vi "Proceed Directory.vi"(8 "error in (no error)":errorcluster, 9 "path":path, 10 "Load Image Report":bool, 11 "Launch File Viewer in":refnum<class "HIJ Vision File Viewer App.lvclass">) -> (0 "error out":errorcluster, 3 "Launch File Viewer out":refnum<class "HIJ Vision File Viewer App.lvclass">)   [LabVIEW 2014, in "HIJ Vision File Viewer App.lvlib" / "HIJ Vision File Viewer App.lvclass"]
uses:
  HIJ Vision File Viewer App.lvclass
  HIJ Vision File Viewer App.lvclass/HIJ Vision File Viewer App.ctl
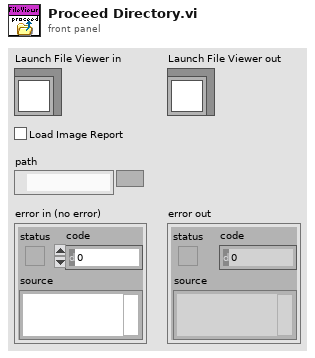
[diagram p1: front panel]
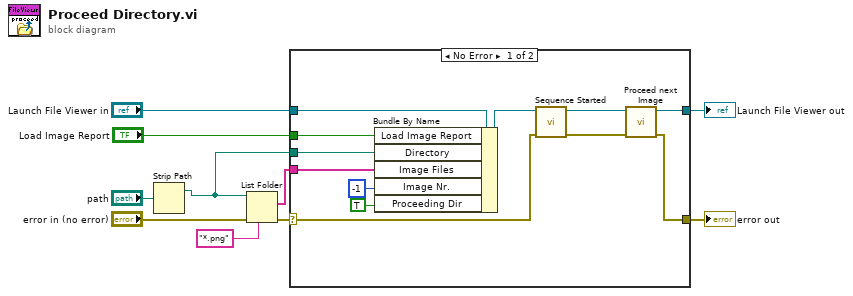
[diagram p0: block diagram]
diagram:
  n1 = Strip Path(path="path") -> (stripped path=w1:path)  [unwired: 1 out]
  n2 = List Folder(path=w1, pattern="*.png", error in="error in (no error)") -> (filenames=w5:string[], error out=w4:errorcluster)  [unwired: 1 in, 2 out]
  n3 = case shown="No Error" w4 {
    selector: w4 -> [w12 w23]
    tunnel: "Launch File Viewer in" -> [w22 w24]
    tunnel: [w16 w24] -> w8
    tunnel: w5 -> [w21 _]
    tunnel: "Load Image Report" -> [w14 _]
    tunnel: [w15 w23] -> w2
    tunnel: w1 -> [w18 _]
    frame No Error {
      n4 = Bundle By Name(cluster=w22, "Load Image Report"=w14, "Directory"=w18, "Image Files"=w21, "Image Nr."=-1, "Proceeding Dir"=TRUE) -> (w17:refnum<class "HIJ Vision File Viewer App.lvclass">)
      n5 = call-dynamic "Sequence Started.vi"("error in (no error)"=w12, "HIJ Vision Application in"=w17) -> ("error out"=w11:errorcluster, "HIJ Vision Application out"=w13:refnum<class "HIJ Vision File Viewer App.lvclass">)  [unwired: 8 in]
      n6 = call-dynamic "Proceed next Image.vi"("error in (no error)"=w11, "Launch File Viewer in"=w13) -> ("error out"=w15:errorcluster, "Launch File Viewer out"=w16:refnum<class "HIJ Vision File Viewer App.lvclass">)  [unwired: 8 in]
    }
    frame Error {
    }
  }
  "error out" <- w2
  "Launch File Viewer out" <- w8
